vi "Zad2_kolokwium.vi"() -> ()   [LabVIEW 2012]
panel:
  in  "Ciśnienie krwi rozkurczowe (mm Hg)":dbl(knob) scale=60.0..130.0
  out "Twoja temperatura i ciśnienie":string
  in  "Ciśnienie krwi skurczowe (mm Hg)":dbl(knob) scale=90.0..200.0
  in  "Temperatura ciała człowieka":dbl(slide) scale=32.0..44.0
  # "Program odczytuje wartość teperatury ciała człowieka z wirtualnego termometru i ciśnienei krwi z wirtualnych manometrów"
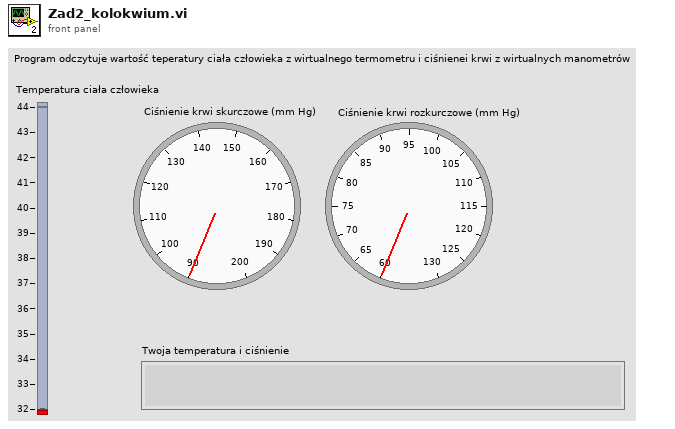
[diagram p1: front panel]
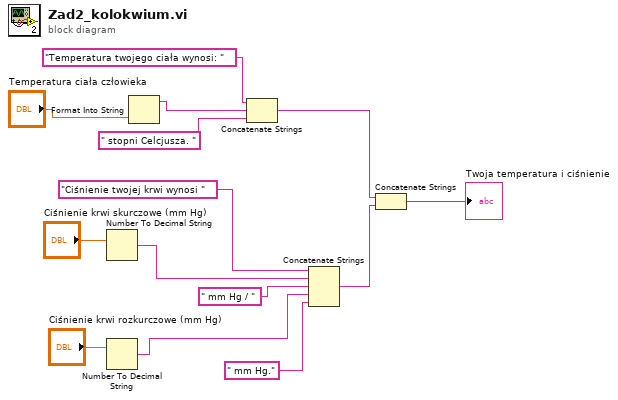
[diagram p0: block diagram]
diagram:
  n1 = Number To Decimal String(number="Ciśnienie krwi skurczowe (mm Hg)") -> (decimal integer string=w3:string)  [unwired: 1 in]
  n2 = Number To Decimal String(number="Ciśnienie krwi rozkurczowe (mm Hg)") -> (decimal integer string=w1:string)  [unwired: 1 in]
  n3 = Format Into String("Temperatura ciała człowieka") -> (resulting string=w12:string)  [unwired: 3 in, 1 out]
  n4 = Concatenate Strings("Temperatura twojego ciała wynosi: ", w12, " stopni Celcjusza. ") -> (w8:string)
  n5 = Concatenate Strings("Ciśnienie twojej krwi wynosi ", w3, " mm Hg / ", w1, " mm Hg.") -> (w7:string)
  n6 = Concatenate Strings(w8, w7) -> (→"Twoja temperatura i ciśnienie":string)
